vi "MainTester.vi"() -> ()   [LabVIEW 2015]
uses:
  <vilib>/Rock Robotics/WPI/SerialPort/WPI_SerialPortRef.ctl
  <vilib>/Rock Robotics/WPI/SerialPort/WPI_SerialPort.ctl
  Old code/packet types.ctl
panel:
  out "Scaled Voltage":dbl
  out "ADC raw values":u32[](array[numeric]) format="%012b"
  out "SerialPortRef 4":T1
  in  "B 2":dbl(slide) scale=0.0..255.0
  in  "G 2":dbl(slide) scale=0.0..255.0
  in  "R 2":dbl(slide) scale=0.0..255.0
  in  "B":dbl(slide) scale=0.0..255.0
  in  "G":dbl(slide) scale=0.0..255.0
  in  "R":dbl(slide) scale=0.0..255.0
  out "SerialPortRef 6":T1
  out "error out 8":errorcluster
  out "SerialPortRef":T1
  out "error out 7":errorcluster
  in  "Close File 2":bool
  in  "Close File":bool
  in  "Display string":string
  out "error out 6":errorcluster
  out "SerialPortRef 5":T1
  out "ADC voltages":dbl[](array[numeric])
  out "error out 4":errorcluster
  out "SerialPortRef 3":T1
  out "error out 3":errorcluster
  out "SerialPortRef 2":T1
  out "error out 2":errorcluster
  out "All Digital Input Vals":bool[](array[boolean])
  out "error out":errorcluster
  in  "stop":bool
  in  "error in (no error)":errorcluster
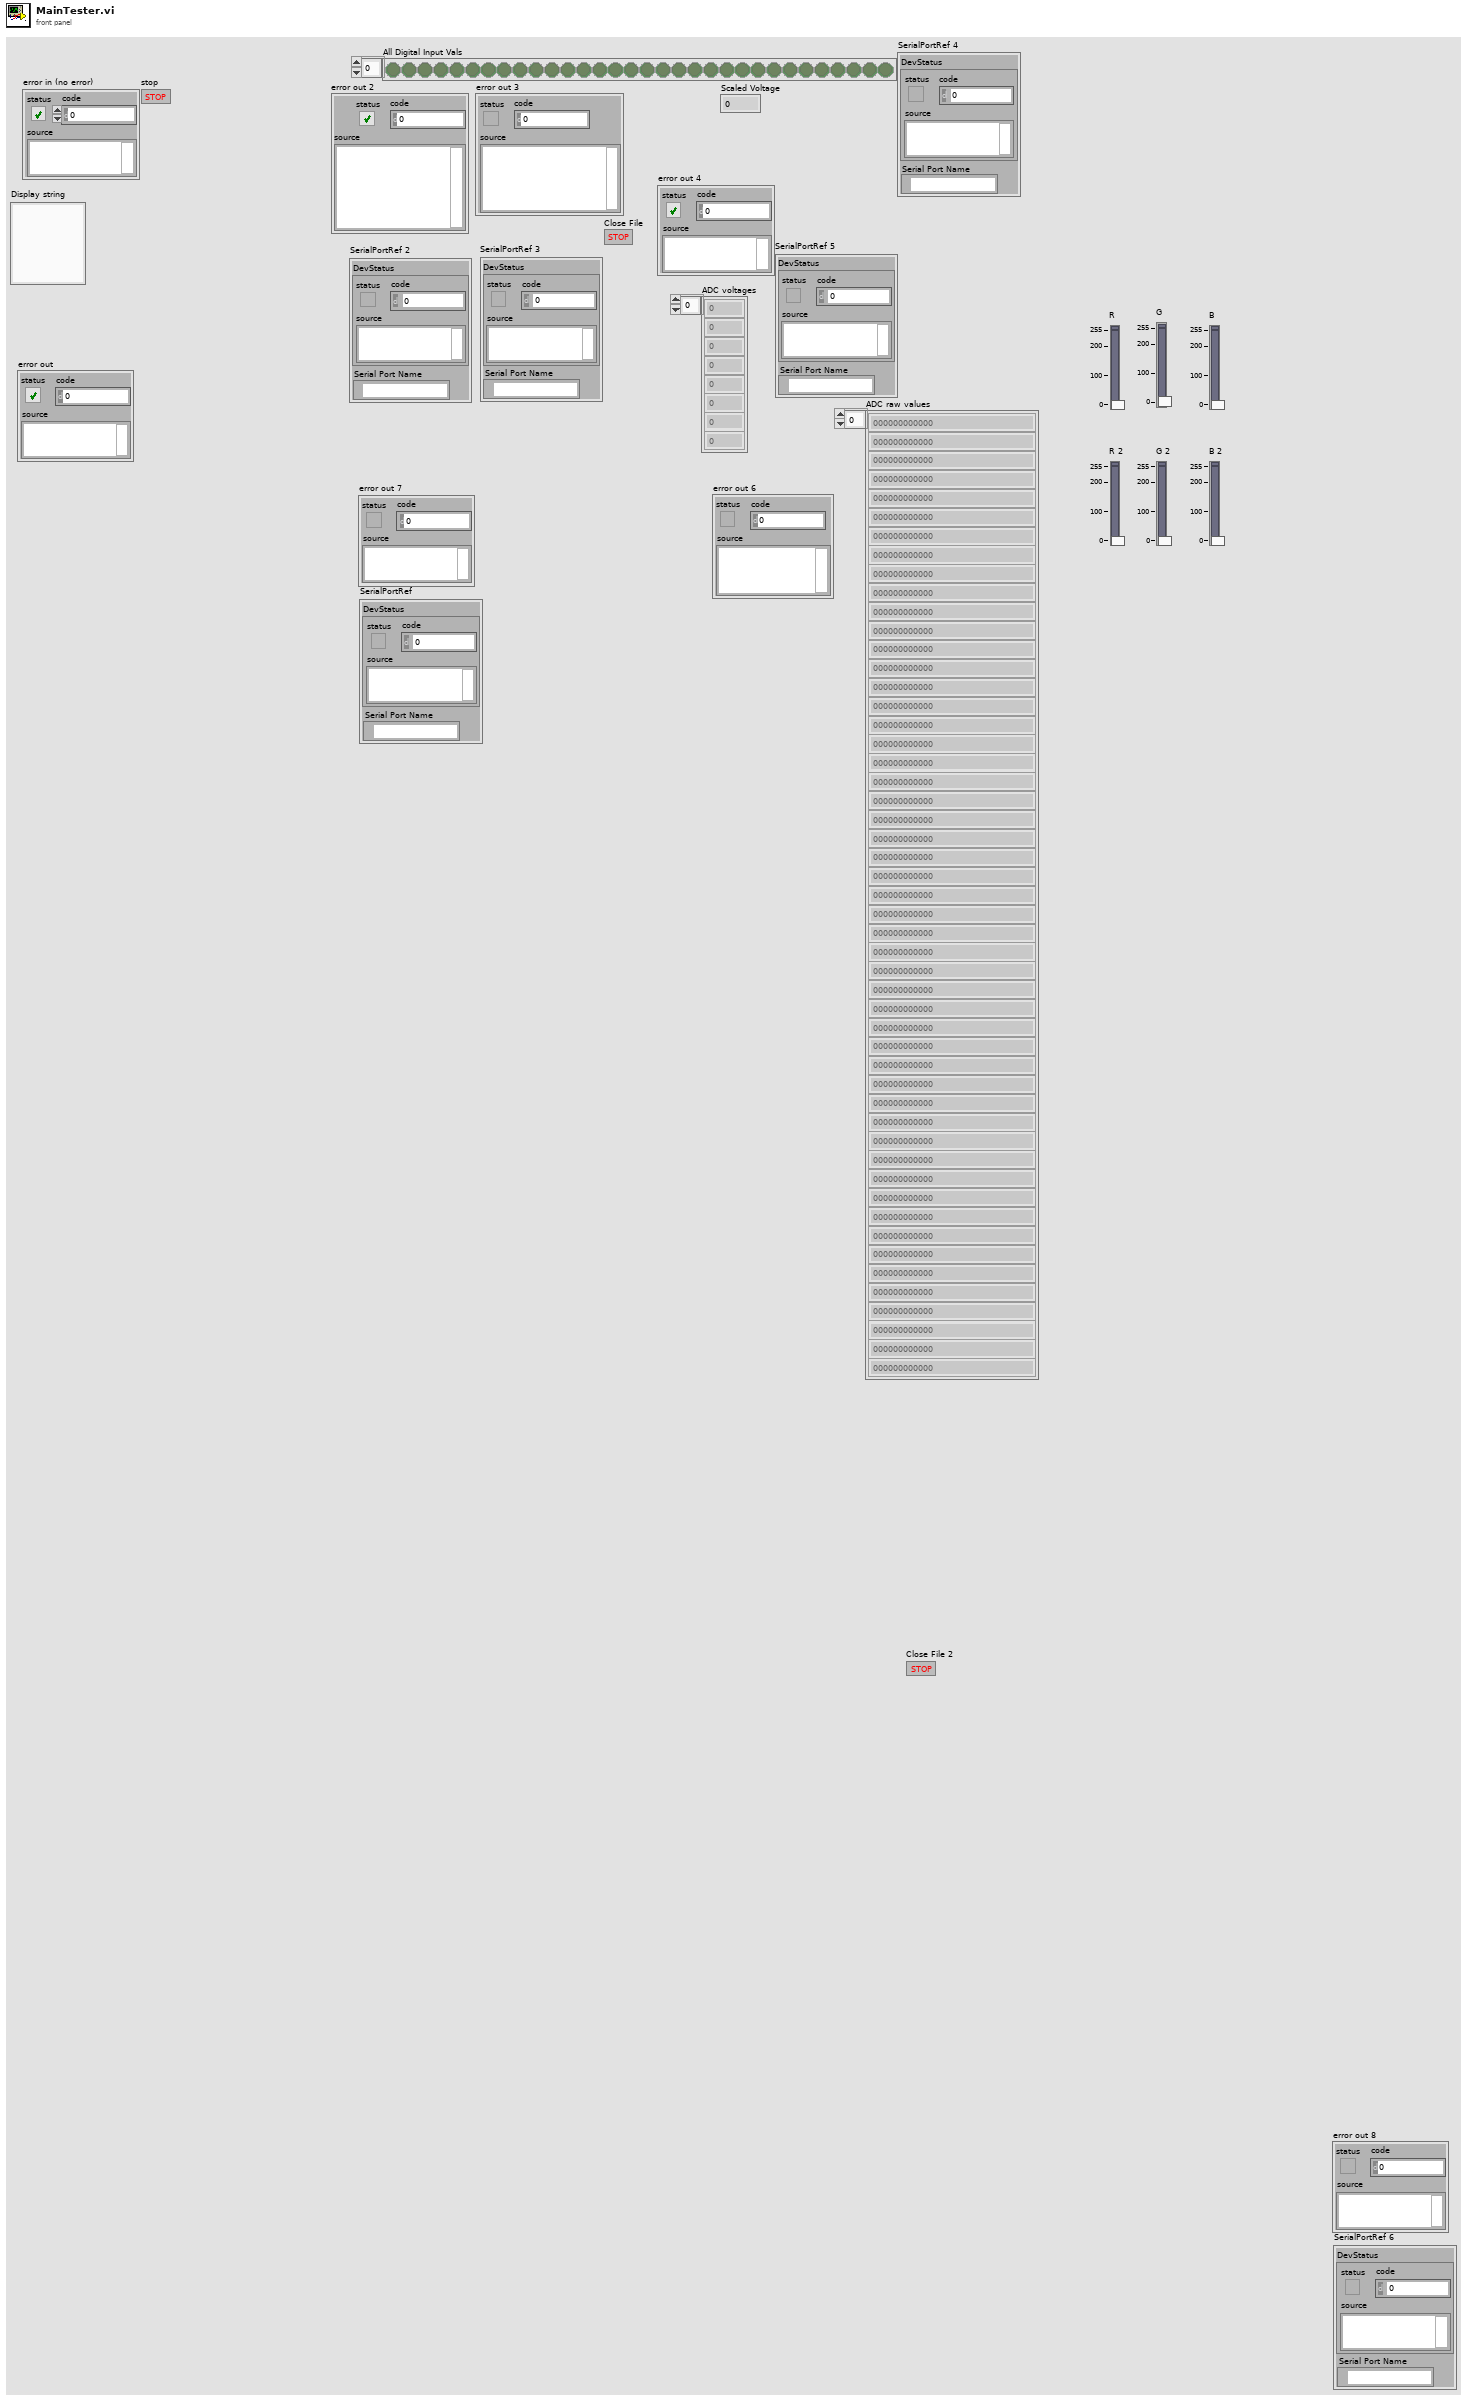
[diagram p1: front panel]
types:
  T1 = typedef "WPI_SerialPortRef.ctl" = cluster{"DevStatus":errorcluster, "Serial Port Name":refnum<visa-resource-name>}
  T2 = typedef "WPI_SerialPort.ctl" = enum16{"Onboard RS-232", "MXP TTL"}
  T3 = typedef "packet types.ctl" = enum16{"Log line", "Open File", "Close File", "Send Header", "Set Time", "Send to LCD"}
  T4 = enum16{"Set Custom RGB", "Set Mode", "Set intensity"}
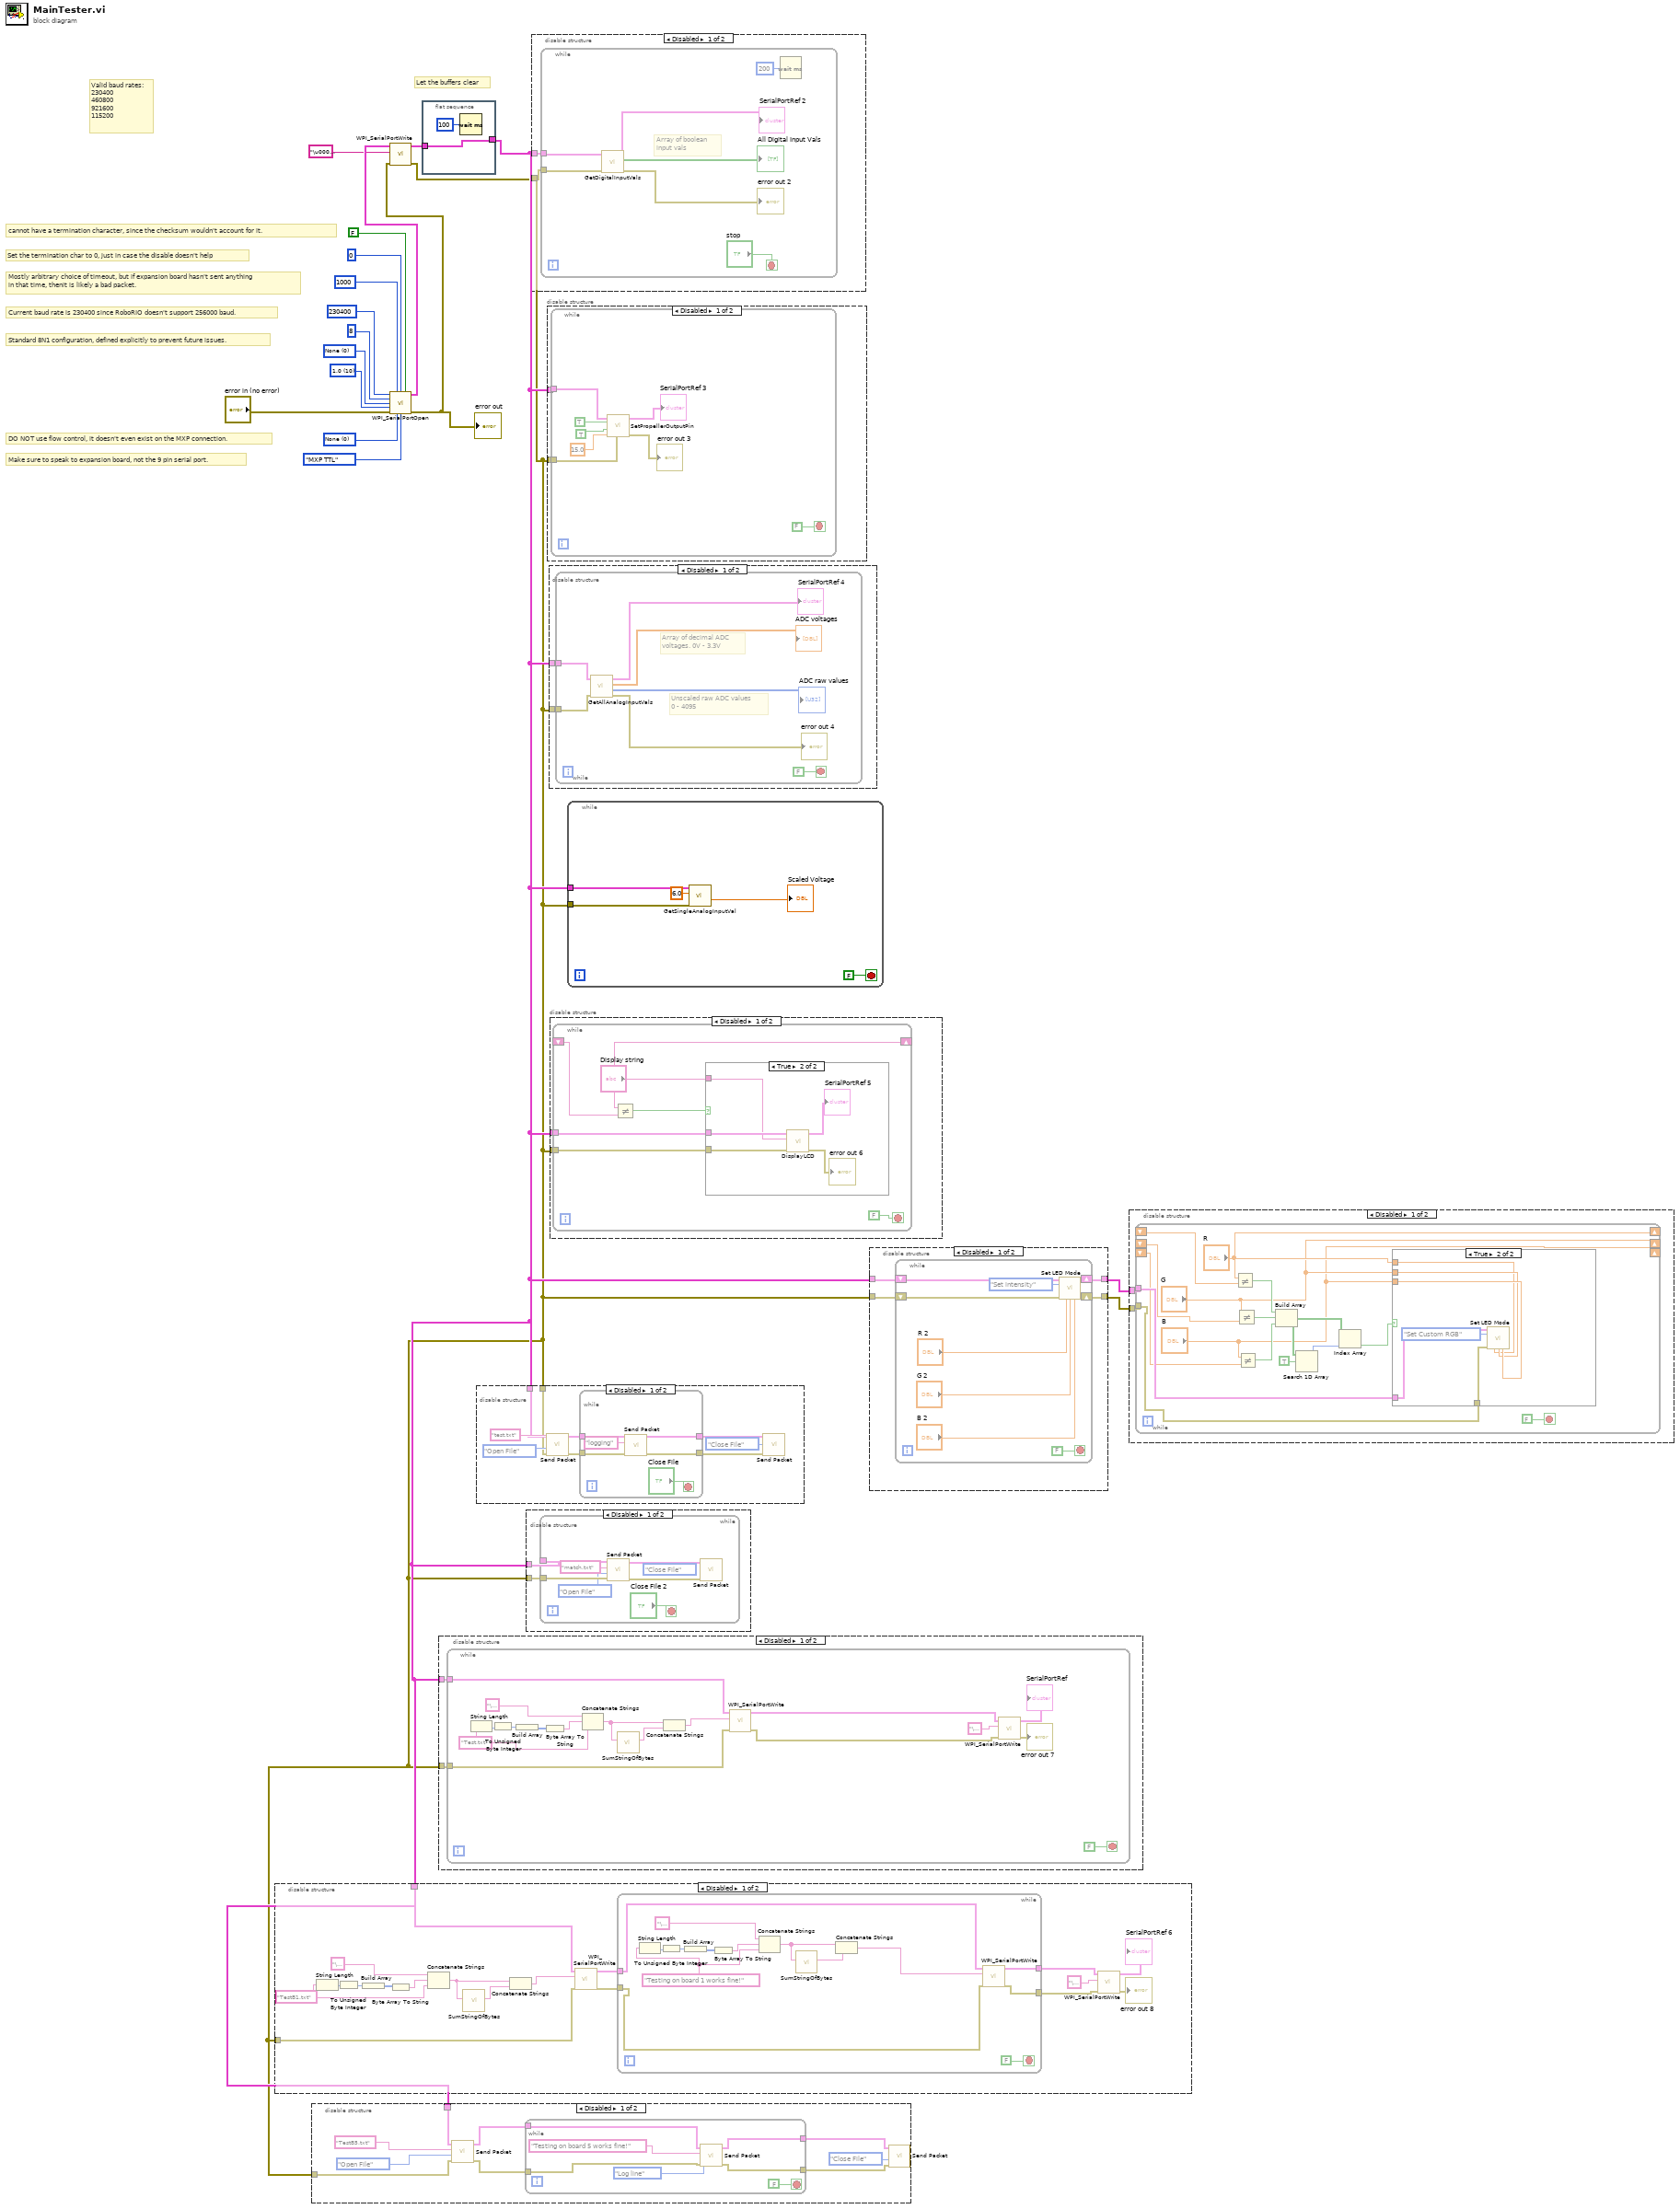
[diagram p0: block diagram]
diagram:
  w17 = u16 10 items=["1.0"=10, "1.5"=15, "2.0"=20] ("Stop Bits")
  w13 = u16 0 items=["None", "XON/XOFF", "RTS/CTS", "XON/XOFF & RTS/CTS", "DTR/DSR", "XON/XOFF & DTR/DSR"] ("Flow Control")
  w12 = u16 0 items=["None", "Odd", "Even", "Mark", "Space"] ("Parity")
  # "Let the buffers clear"
  # "Valid baud rates:\n230400\n460800\n921600\n115200"
  # "Make sure to speak to expansion board, not the 9 pin serial port."
  # "DO NOT use flow control, it doesn't even exist on the MXP connection."
  # "Standard 8N1 configuration, defined explicitly to prevent future issues."
  # "Current baud rate is 230400 since RoboRIO doesn't support 256000 baud."
  # "Mostly arbitrary choice of timeout, but if expansion board hasn't sent anything\nin that time, thenit is likely a bad packet."
  # "Set the termination char to 0, just in case the disable doesn't help"
  # "cannot have a termination character, since the checksum wouldn't account for it."
  n1 = call <vilib>:"WPI_SerialPortOpen.vi"("Baud Rate"=u32 230400, "Timeout Value (ms)"=u32 1000, "Termination Char (0xA = '\\n' = LF)"=u8 0 ("Termination Char (0xA = '\\n' = LF)"), "Enable Termination Char? (T)"=FALSE, "Data Bits"=u16 8, "Parity"=w12, "Stop Bits"=w17, "error in (no error)"="error in (no error)", "Flow Control"=w13, "Serial Port"=WPI_SerialPort."MXP TTL") -> ("SerialPortRef"=w8:T1, "error out"=w7:errorcluster)  [unwired: 4 in]
  "error out" <- w7
  n2 = call <vilib>:"WPI_SerialPortWrite.vi"("error in (no error)"=w7, "Buffer"="\u0004\u0004", "SerialPortRef"=w8) -> ("error out"=w1:errorcluster, "SerialPortRef"=w5:T1)  [unwired: 6 in, 1 out]
  n3 = disable-structure shown="Disabled" {
    disable-tunnel: w2 -> [w20 _]
    disable-tunnel: w1 -> [w19 _]
    frame Disabled {
      w21 = "TestB1.txt"
      n4 = String Length(string=w21) -> (length=w29:i32)
      n5 = To Unsigned Byte Integer(number=w29) -> (unsigned 8bit integer=w32:u8)
      n6 = Build Array(w32) -> (w31:u8[])
      n7 = Byte Array To String(unsigned byte array=w31) -> (string=w30:string)
      n8 = Concatenate Strings("\u0003", w30, w21) -> (w35:string)
      n9 = call "SumStringOfBytes.vi"("String Of Bytes"=w35) -> ("SumAsString"=w36:string)  [unwired: 10 in]
      n10 = Concatenate Strings(w35, w36) -> (w33:string)
      n11 = call <vilib>:"WPI_SerialPortWrite.vi"("error in (no error)"=w19, "Buffer"=w33, "SerialPortRef"=w20) -> ("error out"=w27:errorcluster, "SerialPortRef"=w28:T1)  [unwired: 6 in, 1 out]
      n12 = while {
        tunnel: w28 -> [w50]
        tunnel: w27 -> [w49]
        tunnel: [w39] -> w23
        tunnel: [w38] -> w22
        stop <- FALSE stop-if-true
        w43 = "Testing on board 1 works fine!"
        n13 = String Length(string=w43) -> (length=w45:i32)
        n14 = To Unsigned Byte Integer(number=w45) -> (unsigned 8bit integer=w47:u8)
        n15 = Build Array(w47) -> (w46:u8[])
        n16 = Byte Array To String(unsigned byte array=w46) -> (string=w44:string)
        n17 = Concatenate Strings("\u0001", w44, w43) -> (w41:string)
        n18 = call "SumStringOfBytes.vi"("String Of Bytes"=w41) -> ("SumAsString"=w42:string)  [unwired: 10 in]
        n19 = Concatenate Strings(w41, w42) -> (w40:string)
        n20 = call <vilib>:"WPI_SerialPortWrite.vi"("error in (no error)"=w49, "Buffer"=w40, "SerialPortRef"=w50) -> ("error out"=w38:errorcluster, "SerialPortRef"=w39:T1)  [unwired: 6 in, 1 out]
      }
      n21 = call <vilib>:"WPI_SerialPortWrite.vi"("error in (no error)"=w22, "Buffer"="\u0004", "SerialPortRef"=w23) -> ("error out"=→"error out 8":errorcluster, "SerialPortRef"=→"SerialPortRef 6":T1)  [unwired: 6 in, 1 out]
    }
    frame Enabled {
    }
  }
  n22 = disable-structure shown="Disabled" {
    disable-tunnel: w2 -> [w59 _]
    disable-tunnel: w1 -> [w58 _]
    frame Disabled {
      n23 = call "Send Packet.vi"("error in (no error) 2"=w58, 7:packet_types."Open File", "Log string 2"="TestB5.txt", "SerialPortRef 2"=w59) -> ("error out 2"=w54:errorcluster, "SerialPortRef out 2"=w55:T1)  [unwired: 4 in]
      n24 = while {
        tunnel: w55 -> [w63]
        tunnel: w54 -> [w60]
        tunnel: [w62] -> w52
        tunnel: [w61] -> w51
        stop <- FALSE stop-if-true
        n25 = call "Send Packet.vi"("error in (no error) 2"=w60, 7:packet_types."Log line", "Log string 2"="Testing on board 5 works fine!", "SerialPortRef 2"=w63) -> ("error out 2"=w61:errorcluster, "SerialPortRef out 2"=w62:T1)  [unwired: 4 in]
      }
      n26 = call "Send Packet.vi"("error in (no error) 2"=w51, 7:packet_types."Close File", "SerialPortRef 2"=w52) -> ()  [unwired: 5 in, 2 out]
    }
    frame Enabled {
    }
  }
  n27 = flat-sequence {
    tunnel: [w68] -> w2
    tunnel: w5 -> [w68]
    frame #0 {
      n28 = Wait (ms)(milliseconds to wait=u32 100) -> ()  [unwired: 1 out]
    }
  }
  n29 = disable-structure shown="Disabled" {
    disable-tunnel: w1 -> [w70 _]
    disable-tunnel: w2 -> [w69 _]
    frame Disabled {
      n30 = while {
        tunnel: w69 -> [w87]
        tunnel: w70 -> [w86]
        stop <- FALSE stop-if-true
        w77 = "Test.txt"
        n31 = String Length(string=w77) -> (length=w73:i32)
        n32 = To Unsigned Byte Integer(number=w73) -> (unsigned 8bit integer=w76:u8)
        n33 = Build Array(w76) -> (w75:u8[])
        n34 = Byte Array To String(unsigned byte array=w75) -> (string=w74:string)
        n35 = Concatenate Strings("\u0003", w74, w77) -> (w84:string)
        n36 = call "SumStringOfBytes.vi"("String Of Bytes"=w84) -> ("SumAsString"=w85:string)  [unwired: 10 in]
        n37 = Concatenate Strings(w84, w85) -> (w82:string)
        n38 = call <vilib>:"WPI_SerialPortWrite.vi"("error in (no error)"=w86, "Buffer"=w82, "SerialPortRef"=w87) -> ("error out"=w71:errorcluster, "SerialPortRef"=w72:T1)  [unwired: 6 in, 1 out]
        n39 = call <vilib>:"WPI_SerialPortWrite.vi"("error in (no error)"=w71, "Buffer"="\u0004", "SerialPortRef"=w72) -> ("error out"=→"error out 7":errorcluster, "SerialPortRef"=→"SerialPortRef":T1)  [unwired: 6 in, 1 out]
      }
    }
    frame Enabled {
    }
  }
  n40 = disable-structure shown="Disabled" {
    disable-tunnel: w2 -> [w89 _]
    disable-tunnel: w1 -> [w88 _]
    frame Disabled {
      n41 = call "Send Packet.vi"("error in (no error) 2"=w88, 7:packet_types."Open File", "Log string 2"="test.txt" ("Log string"), "SerialPortRef 2"=w89) -> ("error out 2"=w93:errorcluster, "SerialPortRef out 2"=w94:T1)  [unwired: 4 in]
      n42 = while {
        tunnel: w94 -> [w102]
        tunnel: w93 -> [w101]
        tunnel: [w98] -> w92
        tunnel: [w97] -> w91
        stop <- "Close File" stop-if-true
        n43 = call "Send Packet.vi"("error in (no error) 2"=w101, "Log string 2"="logging" ("Log string"), "SerialPortRef 2"=w102) -> ("error out 2"=w97:errorcluster, "SerialPortRef out 2"=w98:T1)  [unwired: 5 in]
      }
      n44 = call "Send Packet.vi"("error in (no error) 2"=w91, 7:packet_types."Close File", "SerialPortRef 2"=w92) -> ()  [unwired: 5 in, 2 out]
    }
    frame Enabled {
    }
  }
  n45 = disable-structure shown="Disabled" {
    disable-tunnel: w2 -> [w104 _]
    disable-tunnel: w1 -> [w103 _]
    frame Disabled {
      n46 = while {
        tunnel: w104 -> [w111]
        tunnel: w103 -> [w110]
        stop <- "Close File 2" stop-if-true
        (unwired) packet_types."Close File"
        n47 = call "Send Packet.vi"("error in (no error) 2"=w110, 7:packet_types."Open File", "Log string 2"="match.txt" ("Log string"), "SerialPortRef 2"=w111) -> ("error out 2"=w105:errorcluster, "SerialPortRef out 2"=w106:T1)  [unwired: 4 in]
        n48 = call "Send Packet.vi"("error in (no error) 2"=w105, "SerialPortRef 2"=w106) -> ()  [unwired: 6 in, 2 out]
      }
    }
    frame Enabled {
    }
  }
  n49 = disable-structure shown="Disabled" {
    disable-tunnel: w2 -> [w113 _]
    disable-tunnel: w1 -> [w112 _]
    frame Disabled {
      n50 = while {
        tunnel: w112 -> [w118]
        tunnel: w113 -> [w119]
        stop <- "stop" stop-if-true
        # "Array of boolean \ninput vals"
        n51 = call "GetDigitalInputVals.vi"("error in (no error)"=w118, "SerialPortRef"=w119) -> ("error out"=→"error out 2":errorcluster, "All Digital Input Vals"=→"All Digital Input Vals":bool[], "SerialPortRef 2"=→"SerialPortRef 2":T1)  [unwired: 7 in]
        n52 = Wait (ms)(milliseconds to wait=u32 200) -> ()  [unwired: 1 out]
      }
    }
    frame Enabled {
    }
  }
  n53 = disable-structure shown="Disabled" {
    disable-tunnel: w2 -> [w122 _]
    disable-tunnel: w1 -> [w121 _]
    frame Disabled {
      n54 = while {
        tunnel: w121 -> [w127]
        tunnel: w122 -> [w124]
        stop <- FALSE stop-if-true
        n55 = call "SetPropellerOutputPin.vi"("error in (no error)"=w127, "Pin Number"=15.0, "Value"=TRUE, "Dir"=TRUE, "SerialPortRef"=w124) -> ("error out"=→"error out 3":errorcluster, "SerialPortRef 2"=→"SerialPortRef 3":T1)  [unwired: 5 in]
      }
    }
    frame Enabled {
    }
  }
  n56 = disable-structure shown="Disabled" {
    disable-tunnel: w2 -> [w132 _]
    disable-tunnel: w1 -> [w131 _]
    frame Disabled {
      n57 = while {
        tunnel: w132 -> [w139]
        tunnel: w131 -> [w138]
        stop <- FALSE stop-if-true
        # "Unscaled raw ADC values \n0 - 4095"
        # "Array of decimal ADC \nvoltages. 0V - 3.3V"
        n58 = call "GetAllAnalogInputVals.vi"("error in (no error)"=w138, "SerialPortRef"=w139) -> ("error out"=→"error out 4":errorcluster, "ADC raw values"=→"ADC raw values":u32[], "ADC voltages"=→"ADC voltages":dbl[], "SerialPortRef 2"=→"SerialPortRef 4":T1)  [unwired: 6 in]
      }
    }
    frame Enabled {
    }
  }
  n59 = disable-structure shown="Disabled" {
    disable-tunnel: w2 -> [w141 _]
    disable-tunnel: w1 -> [w140 _]
    frame Disabled {
      n60 = while {
        tunnel: w141 -> [w145]
        tunnel: w140 -> [w147]
        shift-right: ["Display string"] -> _
        shift-left: _ -> [w143]
        stop <- FALSE stop-if-true
        n61 = Not Equal?(x="Display string", y=w143) -> (x != y?=w142:bool)
        n62 = case shown="True" w142 {
          tunnel: w145 -> [_ w152]
          tunnel: w147 -> [_ w151]
          tunnel: "Display string" -> [_ w148]
          frame False {
          }
          frame True {
            n63 = call "DisplayLCD.vi"("error in (no error)"=w151, "Display string"=w148, "SerialPortRef"=w152) -> ("error out"=→"error out 6":errorcluster, "SerialPortRef 2"=→"SerialPortRef 5":T1)  [unwired: 7 in]
          }
        }
      }
    }
    frame Enabled {
    }
  }
  n64 = while {
    tunnel: w2 -> [w157]
    tunnel: w1 -> [w156]
    stop <- FALSE stop-if-true
    n65 = call "GetSingleAnalogInputVal.vi"("error in (no error)"=w156, "Pin number 0-7"=6.0, "SerialPortRef"=w157) -> ("Scaled Voltage"=→"Scaled Voltage":dbl)  [unwired: 5 in, 3 out]
  }
  n66 = disable-structure shown="Disabled" {
    disable-tunnel: w1 -> [w161 _]
    disable-tunnel: w2 -> [w160 _]
    disable-tunnel: [w159 _] -> w4
    disable-tunnel: [w158 _] -> w3
    frame Disabled {
      n67 = while {
        shift-right: [w167] -> w158
        shift-left: w161 -> [w170]
        shift-right: [w168] -> w159
        shift-left: w160 -> [w169]
        stop <- FALSE stop-if-true
        n68 = call "Set LED Mode.vi"("SerialPortRef 3"=w169, 5:T4."Set intensity" ("Enum"), "error in (no error)"=w170, "Red"="R 2", "Green"="G 2", "Blue"="B 2") -> ("SerialPortRef"=w168:T1, "error out"=w167:errorcluster)  [unwired: 8 in]
      }
    }
    frame Enabled {
    }
  }
  n69 = disable-structure shown="Disabled" {
    disable-tunnel: w4 -> [w172 _]
    disable-tunnel: w3 -> [w171 _]
    frame Disabled {
      n70 = while {
        tunnel: w172 -> [w186]
        tunnel: w171 -> [w187]
        shift-right: ["R"] -> _
        shift-left: _ -> [w185]
        shift-right: ["G"] -> _
        shift-left: _ -> [w184]
        shift-right: ["B"] -> _
        shift-left: _ -> [w183]
        stop <- FALSE stop-if-true
        n71 = Not Equal?(x="R", y=w185) -> (x != y?=w180:bool)
        n72 = Not Equal?(x="G", y=w184) -> (x != y?=w182:bool)
        n73 = Not Equal?(x="B", y=w183) -> (x != y?=w181:bool)
        n74 = Build Array(w180, w182, w181) -> (w177:bool[])
        n75 = Search 1D Array(1D array=w177, element=TRUE) -> (index of element=w178:i32)  [unwired: 1 in]
        n76 = Index Array(array=w177, index=w178) -> (element=w176:bool)
        n77 = case shown="True" w176 {
          tunnel: w187 -> [_ w193]
          tunnel: w186 -> [_ w194]
          tunnel: "R" -> [_ w189]
          tunnel: "G" -> [_ w190]
          tunnel: "B" -> [_ w191]
          frame False {
          }
          frame True {
            n78 = call "Set LED Mode.vi"("SerialPortRef 3"=w194, 5:enum16{"Set Custom RGB", "Set Mode"}."Set Custom RGB" ("Enum"), "error in (no error)"=w193, "Red"=w189, "Green"=w190, "Blue"=w191) -> ()  [unwired: 8 in, 2 out]
          }
        }
      }
    }
    frame Enabled {
    }
  }
